vi "YKMW100 Clear Error Display.vi"(0 "VISA session":refnum<visa-resource-name>="MW100", 9 "Timeout (25000)":u32=100, 11 "error in (no error)":errorcluster, 13 "Source (\"\")":string) -> (4 "dup VISA session":refnum<visa-resource-name>, 7 "Send Message (\"\")":string="CE0", 8 "Read Buffer":string, 15 "error out":errorcluster)   [LabVIEW 2023]
doc: "This VI sends the message. Then it returns the response."
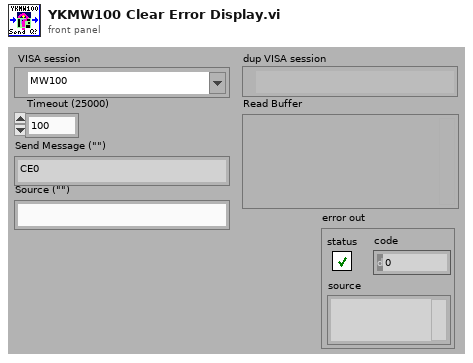
[diagram p1: front panel]
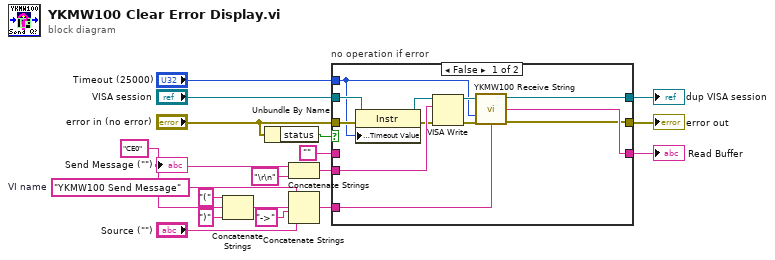
[diagram p0: block diagram]
diagram:
  w2 = "CE0" ("Send Message (\"\")")
  w6 = "YKMW100 Send Message"  # VI name
  n1 = Concatenate Strings("(", w2, ")") -> (w7:string)
  n2 = Unbundle By Name("error in (no error)") -> ("status"=w13:bool)
  n3 = Concatenate Strings(w2, "\r\n") -> (w17:string)
  n4 = Concatenate Strings(w6, w7, "->", "Source (\"\")") -> (w12:string)
  n5 = case "no operation if error" shown="False" w13 {
    tunnel: "VISA session" -> [w27 w33]
    tunnel: w17 -> [w30 _]
    tunnel: [w21 w33] -> w4
    tunnel: [w19 w32] -> w18
    tunnel: "error in (no error)" -> [w29 w32]
    tunnel: w12 -> [w23 _]
    tunnel: "Timeout (25000)" -> [w22 _]
    tunnel: [w20 w31] -> w5
    tunnel: "" -> [_ w31]
    frame False {
      n6 = property class="Instr"(reference=w27, error in=w29, "General Settings:Timeout Value"=w22) -> (reference out=w26:refnum<visa-resource-name>, error out=w28:errorcluster)
      n7 = VISA Write(VISA resource name=w26, write buffer=w30, error in (no error)=w28) -> (VISA resource name out=w25:refnum<visa-resource-name>, error out=w24:errorcluster)  [unwired: 1 out]
      n8 = call "YKMW100 Receive String.vi"("VISA session"=w25, "Timeout (25000)"=w22, "error in (no error)"=w24, "Source (\"\")"=w23) -> ("dup VISA session"=w21:refnum<visa-resource-name>, "Read Buffer"=w20:string, "error out"=w19:errorcluster)  [unwired: 9 in]
    }
    frame True {
    }
  }
  "error out" <- w18
  "dup VISA session" <- w4
  "Read Buffer" <- w5
  "Send Message (\"\")" <- w2
